vi "Set Enable State on Multiple Controls.vi"(8 "error in (no error)":errorcluster, 10 "Enable?":bool, 11 "Controls":refnum<vi>[](array[refnum])) -> (0 "error out":errorcluster)   [LabVIEW 2026]
doc: "Sets all the controls in the input array to the \"Enable state\" value."
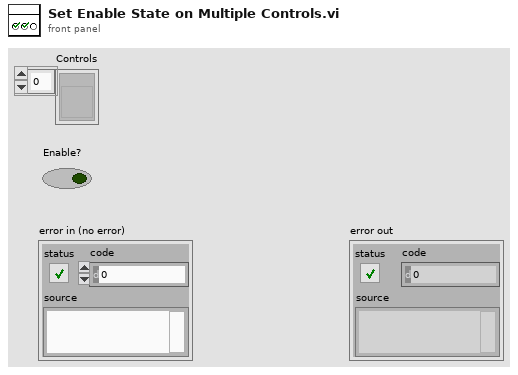
[diagram p1: front panel]
types:
  T1 = enum8{"Enabled", "Disabled", "Disabled and Grayed Out"}
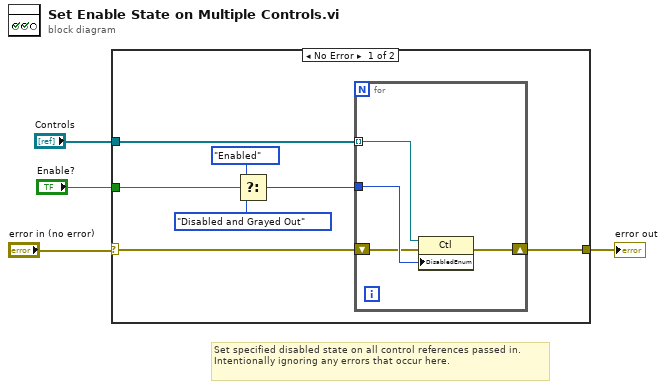
[diagram p0: block diagram]
diagram:
  # "Set specified disabled state on all control references passed in. Intentionally ignoring any errors that occur here."
  n1 = case shown="No Error" "error in (no error)" {
    selector: "error in (no error)" -> [w6 w16]
    tunnel: "Controls" -> [w8 _]
    tunnel: "Enable?" -> [w7 _]
    tunnel: [w5 w16] -> w1
    frame No Error {
      n2 = Select(t=T1."Enabled" ("Disabled"), s=w7, f=T1."Disabled and Grayed Out" ("Disabled")) -> (s? t:f=w11:T1)
      n3 = for {
        tunnel: w8 -> [w15] mode=indexing
        tunnel: w11 -> [w14]
        shift-right: [w12] -> w5
        shift-left: w6 -> [w13]
        n4 = property class="Ctl"(reference=w15, error in=w13, "DisabledEnum"=w14) -> (error out=w12:errorcluster)  [unwired: 1 out]
      }
    }
    frame Error {
    }
  }
  "error out" <- w1
